vi "UI.vi"(0 "reference in":refnum<class "GUI PumpMotor.lvclass">, 5 "error in (no error)":errorcluster) -> (14 "reference out":refnum<class "GUI PumpMotor.lvclass">, 19 "error out":errorcluster)   [LabVIEW 2019, in "GUI PumpMotor.lvclass"]
uses:
  GUI PumpMotor.lvclass
  D:/GIT H4000/H4000/src/GUI_class/GUI.lvclass
  modbus engine custom/MB_ENGINE_class/Engine Alarms.ctl
  modbus engine custom/MB_ENGINE_class/Settings.ctl
  modbus engine custom/MB_ENGINE_class/cmd enum.ctl
  modbus engine custom/MB_ENGINE_class/Engine State.ctl
  TypeDef/Needle Valve Settings.ctl
  GUI_class/GUI.lvclass/GUI.ctl
  TypeDef/Needle Valve Data.ctl
  TypeDef/Needle Valve State.ctl
  modbus engine custom/MB_ENGINE_class/Limits Status.ctl
  SV_Wrap/SharedVariableWrapper.lvclass/SharedVariableWrapper.ctl
  MessageAMC_class/MessageAMC.lvclass
  D:/GIT H4000/H4000/src/MessageInterface_class/MessageInterface.lvclass
  0872259c-c1b7-4622-8eff-96544e628326.vi
  1b4fed76-272f-4eb9-b435-1b7916789d73.vi
  d0ca9bf2-7cd9-4c29-a03d-de1c10393a74.vi
  GUI_class/Set Win State.vi
  GUI_class/protected/GetSheredData.vi
  0872259c-c1b7-4622-8eff-96544e628326.vi/63923c93-3271-404a-8daf-727763f159bc.vi
  SV_Wrap/Write Var Info.vi
  SV_Wrap/Read Var Info.vi
  1b4fed76-272f-4eb9-b435-1b7916789d73.vi/fad6aa2d-1fd6-40e9-9208-cebdd25b163b.vi
  d0ca9bf2-7cd9-4c29-a03d-de1c10393a74.vi/ea186c4c-0445-4979-bfc0-5907181f2b8f.vi
  SV_Wrap/Read connection str.vi
  <userlib>/_OpenG.lib/time/time.llb/Tick Count (ms)__ogtk.vi
  GUI_class/GUI.lvclass
  MessageInterface_class/MessageInterface.lvclass
  SV_Wrap/SharedVariableWrapper.lvclass
  modbus engine custom/MB_ENGINE_class/MB_ENGINE.lvclass
panel:
  in  "Needle Valve Settings":T1={"average size"=0, "open force"=12, "close force"=12, "open settings"={"ACC Steps Per Sec^2"=0, "DEC Steps Per Sec^2"=0, "Min Velosity Step Per Sec"=0, "Max Velosity Step Per Sec"=0, "MicroStep"=0}, "close settings"={"ACC Steps Per Sec^2"=0, "DEC Steps Per Sec^2"=0, "Min Velosity Step Per Sec"=0, "Max Velosity Step Per Sec"=0, "MicroStep"=0}} caption="Settings"
  in  "Engine State":T3 items=["ACCELERATING", "DECELERATINGTOSTOP", "DECELERATING", "STEADY", "INDEX_ACCEL", "NDEX_RUN", "INDEX_DECEL", "INDEX_DWELL", "INACTIVE", "STANDBY", "STANDBYTOINACTIVE"]
  out "String 2":string
  out "String":string
  in  "clear fault":bool
  in  "stop":bool
  in  "close":bool
  in  "open":bool
  in  "Set_cmd":bool
  in  "cmd to write":T4 items=["0 Idle"=0, "1 GoTo Absolute Position"=1, "2 GoTo Relative"=2, "10 GoTo Home Position"=10, "11 Set Home Position"=11, "12 Set FindHome Mode"=12, "13 Reset FindHome Mode"=13, "14 Get FindHome State"=14, "20 Hard Stop"=20, "21 HiZ Stop"=21, "22 Soft Stop"=22, "30 Clear Fault"=30, "40 Encoder Set Home"=40, "70 Driver Init"=70]
  in  "set":bool
  out "Kinematic":T2
  out "Waveform Chart - Dark 3":dbl(graph) caption="Угол"
  out "encoder":i32(graph) caption="Энкодер"
  out "step":i32(graph) caption="ШАГ"
  out "Alarms":T5
  out "DO 19":bool
  out "Connect":bool
  in  "stop":bool
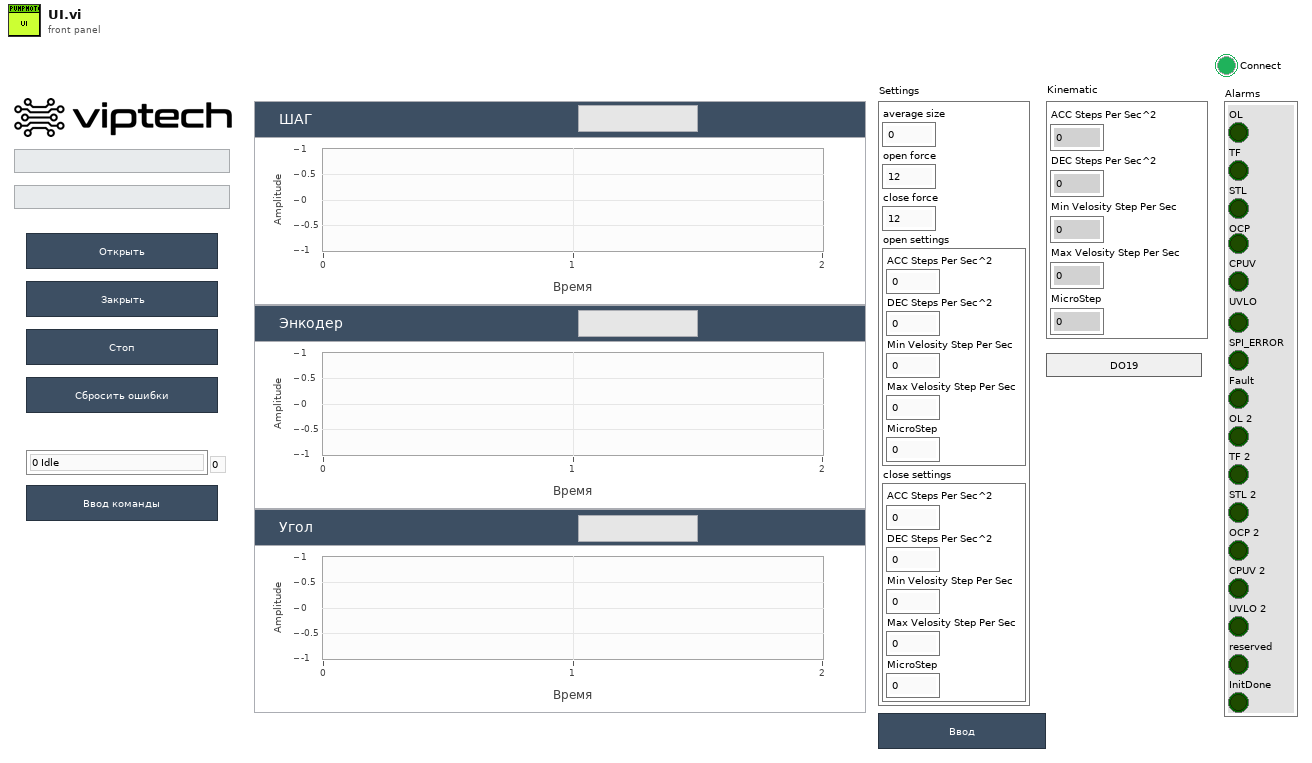
[diagram p1: front panel]
types:
  T1 = typedef "Needle Valve Settings.ctl" = cluster{"average size":i32, "open force":u16, "close force":u16, "open settings":T2, "close settings":T2}
  T2 = typedef "MB_ENGINE.lvclass/Settings.ctl" = cluster{"ACC Steps Per Sec^2":u16, "DEC Steps Per Sec^2":u16, "Min Velosity Step Per Sec":u16, "Max Velosity Step Per Sec":u16, "MicroStep":u16}
  T3 = typedef "MB_ENGINE.lvclass/Engine State.ctl" = u16
  T4 = typedef "MB_ENGINE.lvclass/cmd enum.ctl" = u16
  T5 = typedef "MB_ENGINE.lvclass/Engine Alarms.ctl" = cluster{"OL":bool, "TF":bool, "STL":bool, "OCP":bool, "CPUV":bool, "UVLO":bool, "SPI_ERROR":bool, "Fault":bool, "OL 2":bool, "TF 2":bool, "STL 2":bool, "OCP 2":bool, "CPUV 2":bool, "UVLO 2":bool, "reserved":bool, "InitDone":bool}
  T6 = enum32{"Invalid", "Standard", "Closed", "Hidden", "Minimized", "Maximized"}
  T7 = enum32{"invalid app kind", "Development System", "Run Time System", "Student Edition", "Embedded LabVIEW", "Evaluation", "Custom"}
  T8 = typedef "SharedVariableWrapper.lvclass/Config.ctl" = cluster{"connection str":string, "timeout":dbl, "ip":string}
  T9 = cluster{"Core":cluster{"Current VI Reference":refnum<vi>, "Close Panel on Exit?":bool}, "amc":refnum<class "MessageAMC.lvclass">, "satting name":string, "Needle Valve Settings":T1}
  T10 = cluster{"Current VI Reference":refnum<vi>, "Close Panel on Exit?":bool}
  T11 = typedef "Needle Valve Data.ctl" = cluster{"Engine State":T3, "StateValveModbus":T12, "Alarms":T5, "RAW Possition":i32, "Angele":dbl, "Step":i32, "Encoder":i32, "Kinematic":T2, "Limits":T13}
  T12 = typedef "Needle Valve State.ctl" = enum16{"IDLE", "OPENING", "CLOSING", "STOP"}
  T13 = typedef "MB_ENGINE.lvclass/Limits Status.ctl" = cluster{"Fault 2 Switch":bool, "Fault 1 Switch":bool, "Center(Home)":bool, "Lower Limit":bool, "Upper Limit":bool}
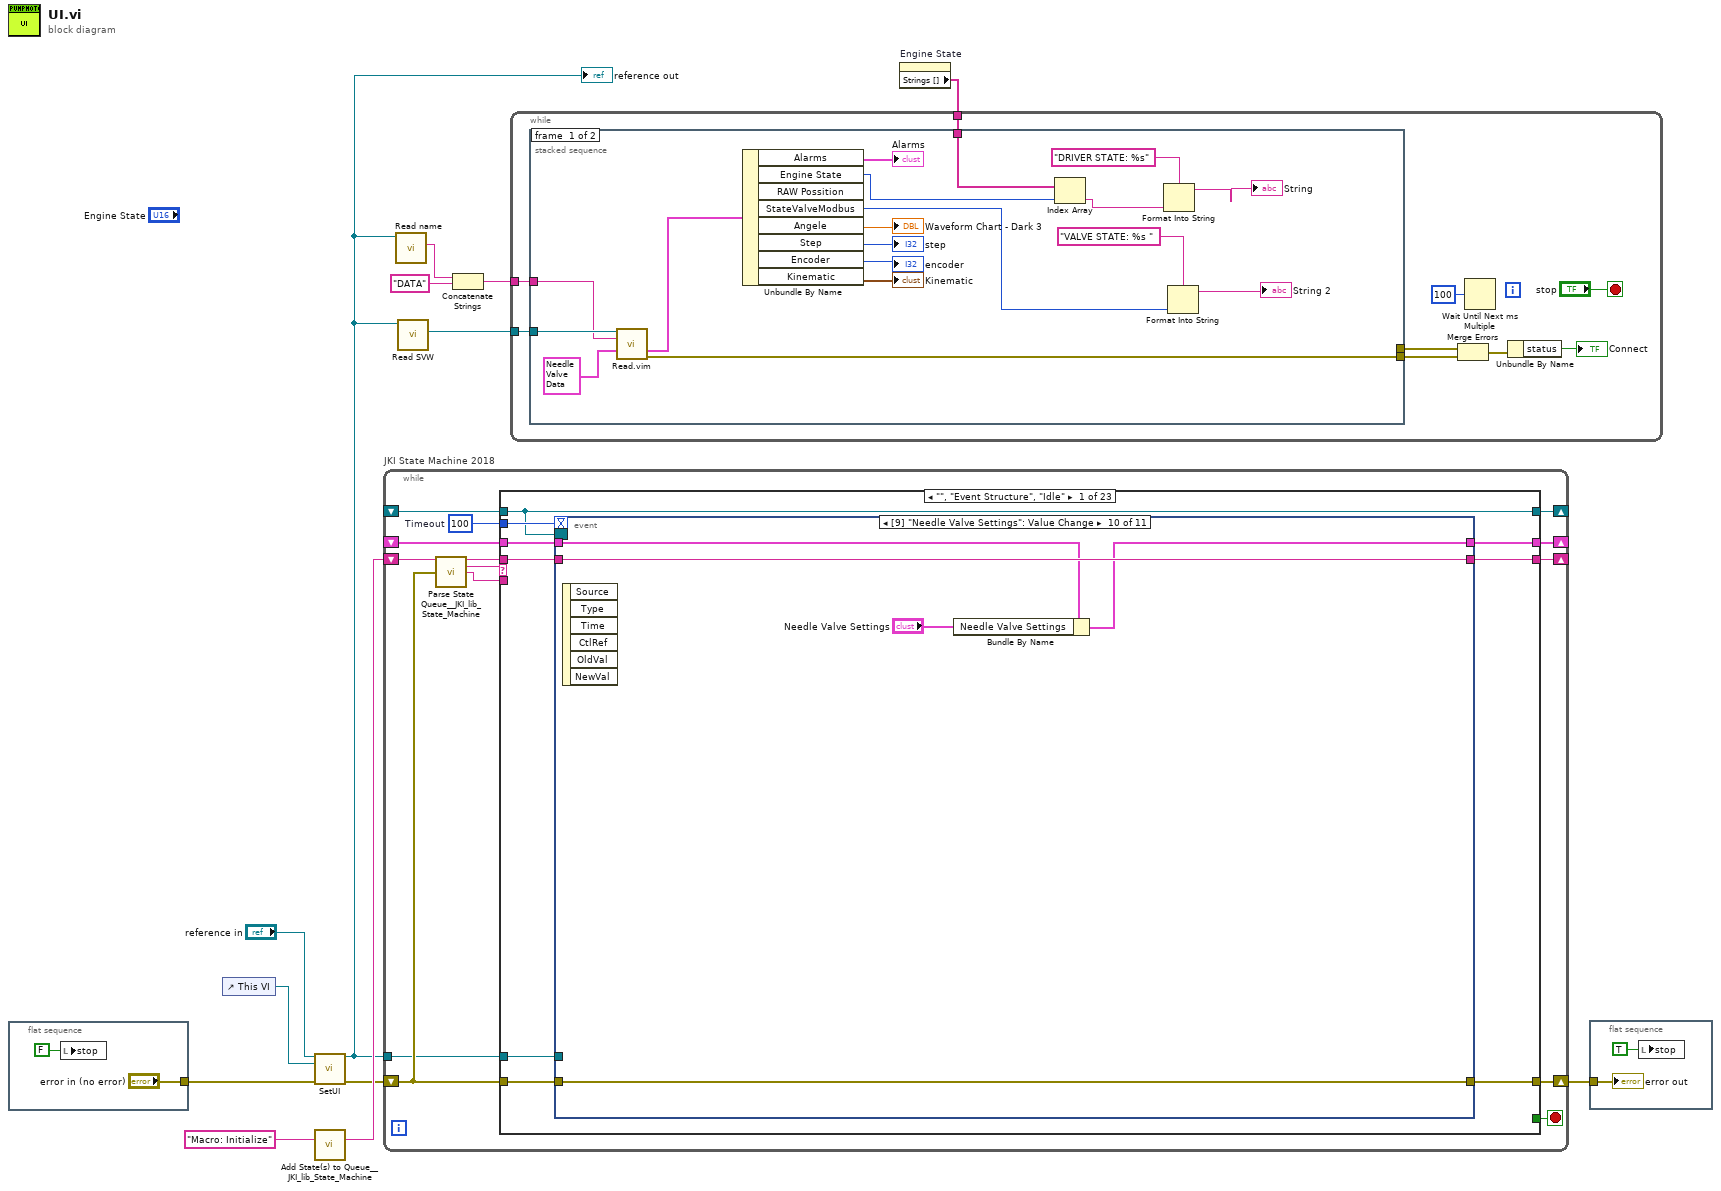
[diagram p0: block diagram]
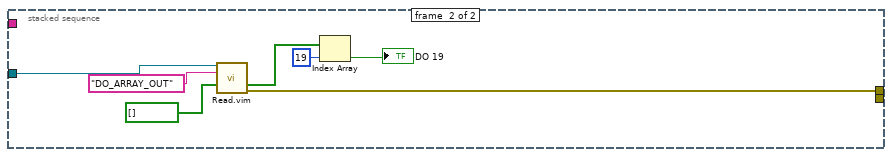
[diagram p2: hidden frame]
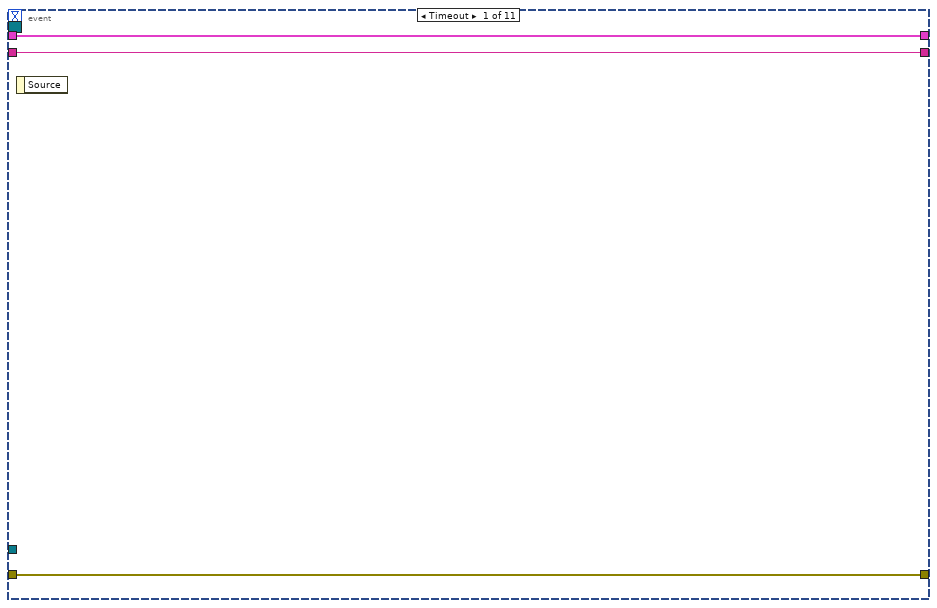
[diagram p3: hidden frame]
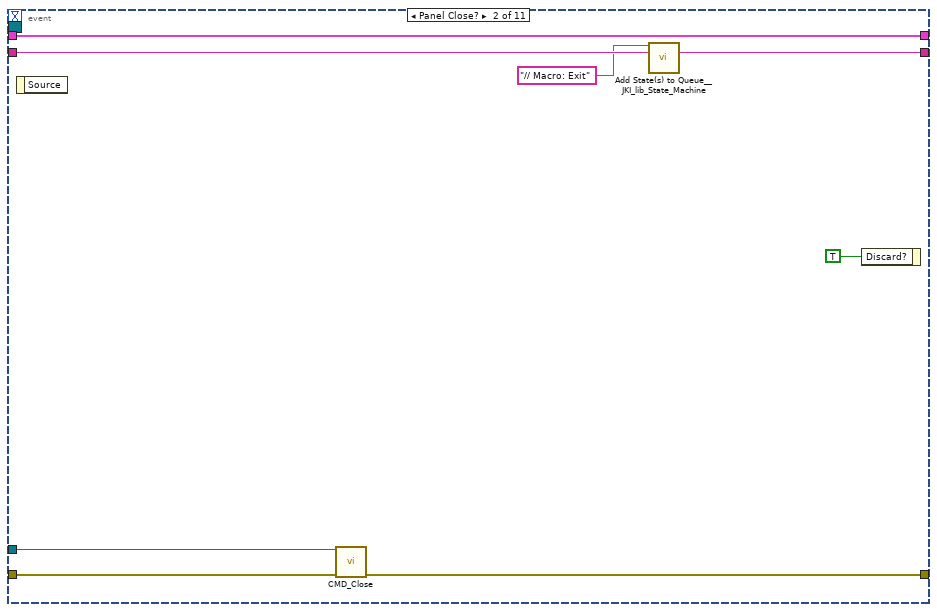
[diagram p4: hidden frame]
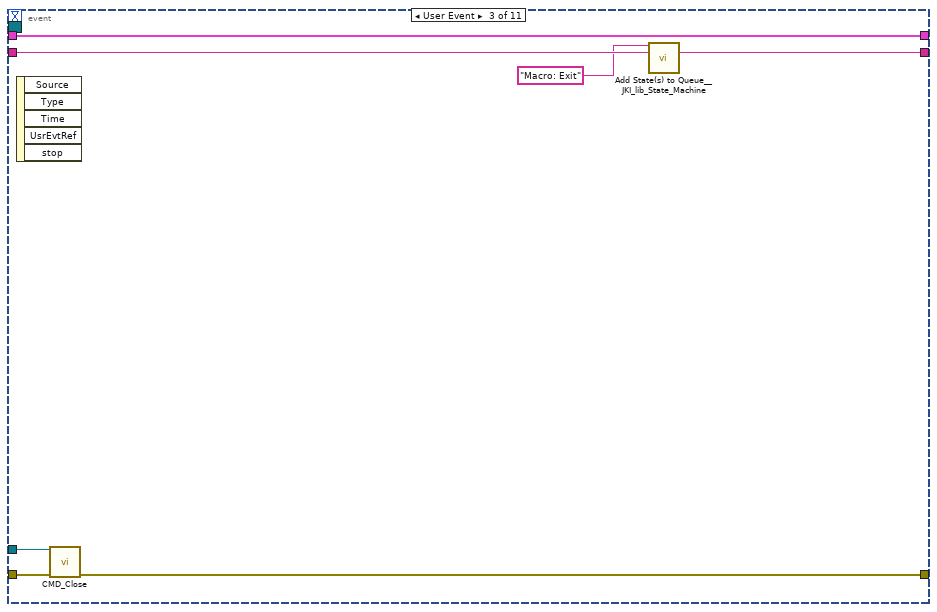
[diagram p5: hidden frame]
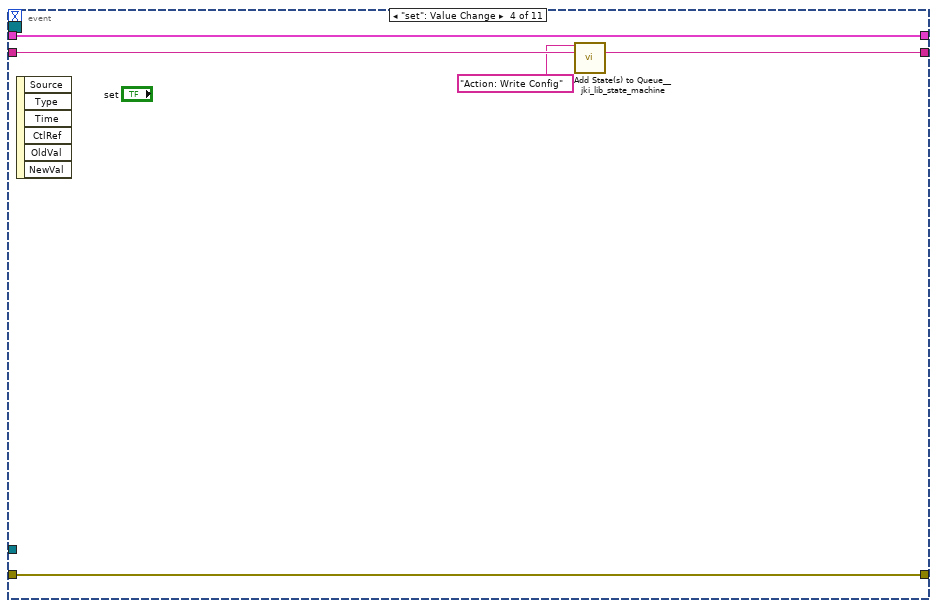
[diagram p6: hidden frame]
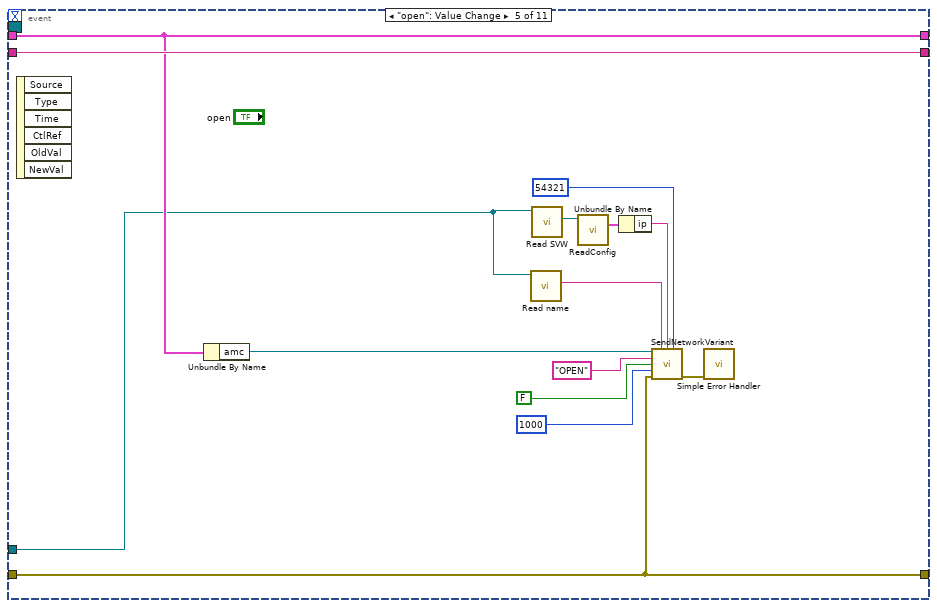
[diagram p7: hidden frame]
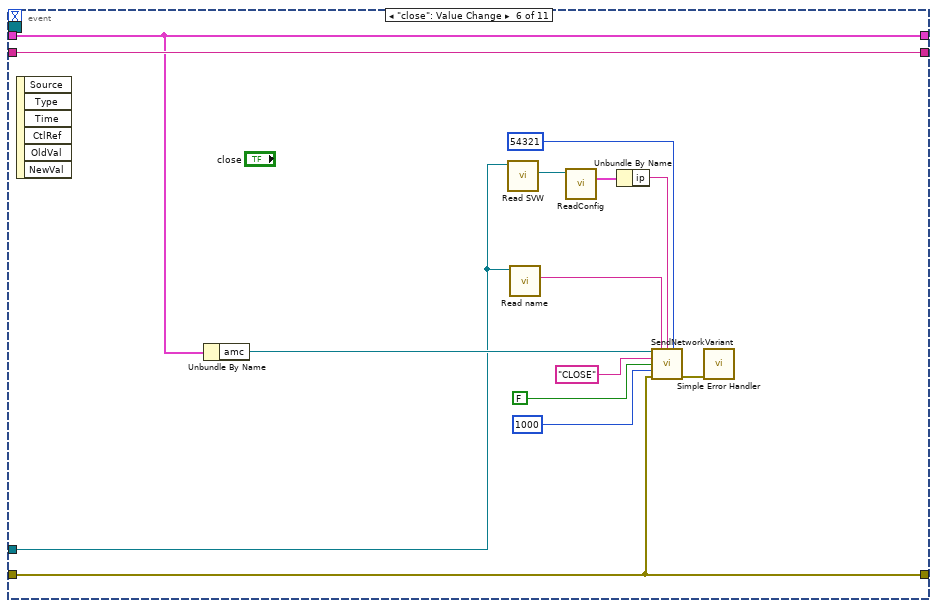
[diagram p8: hidden frame]
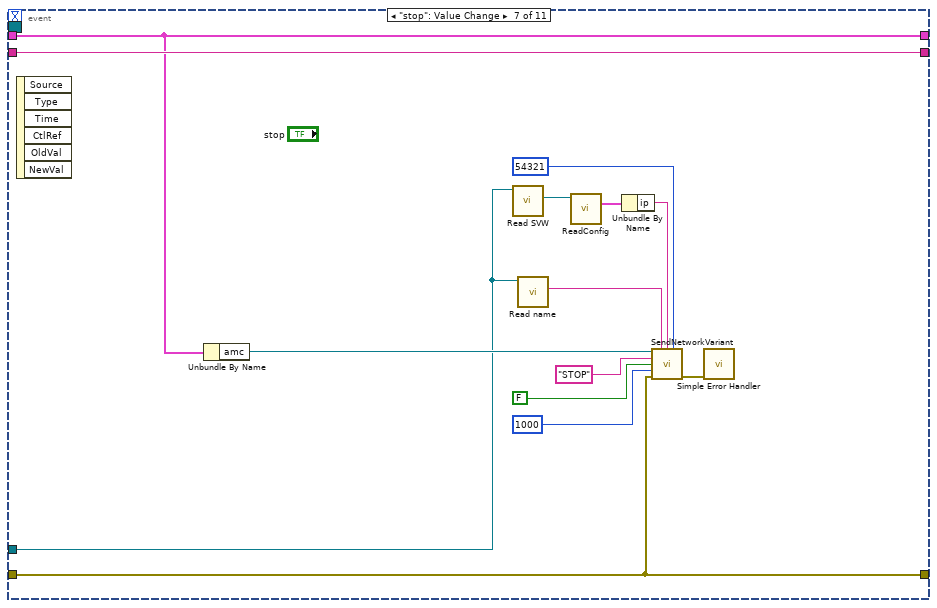
[diagram p9: hidden frame]
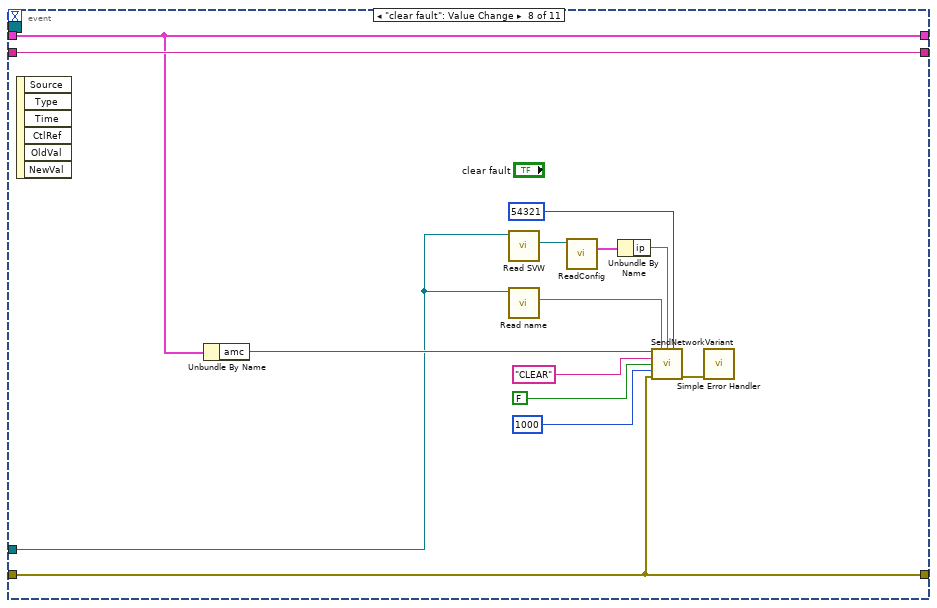
[diagram p10: hidden frame]
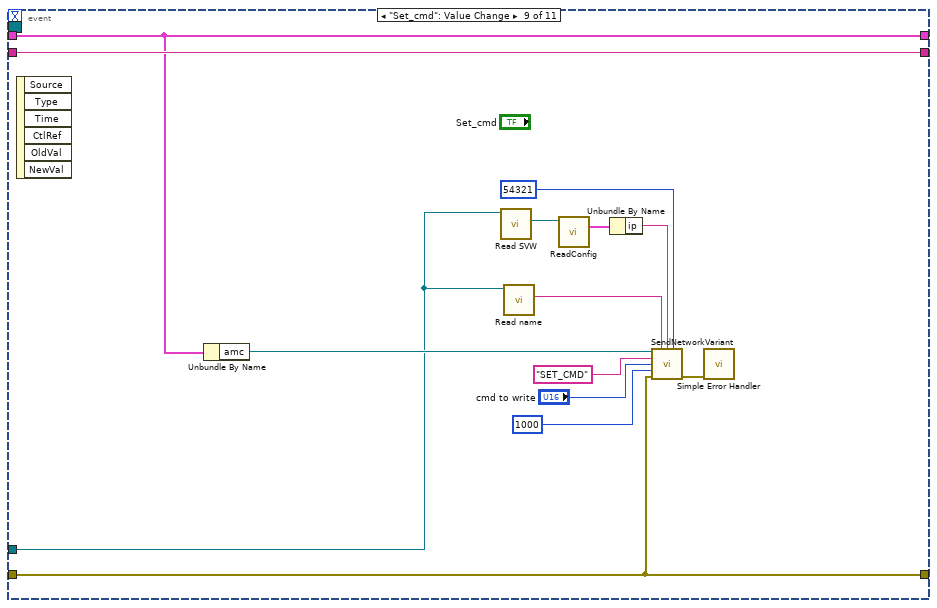
[diagram p11: hidden frame]
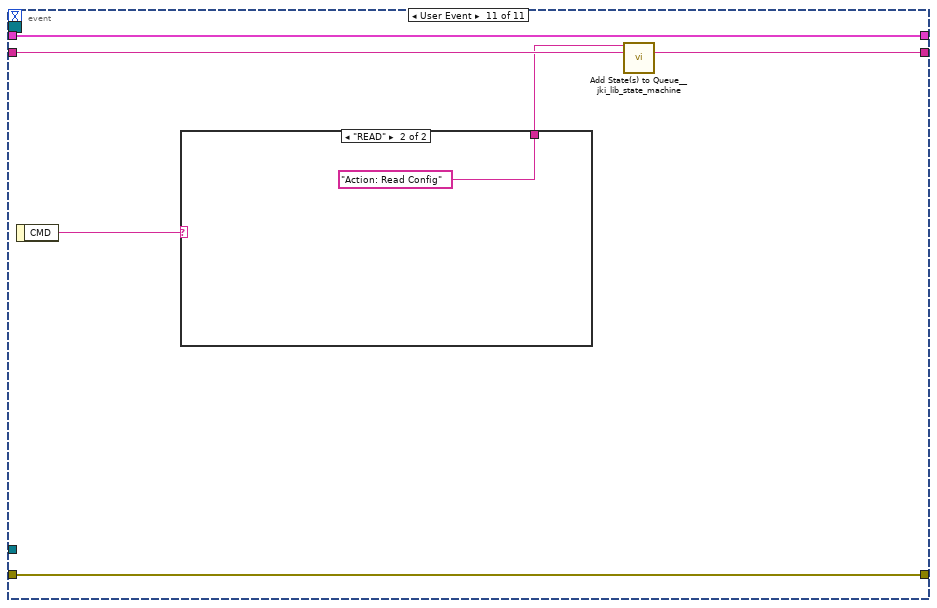
[diagram p12: hidden frame]
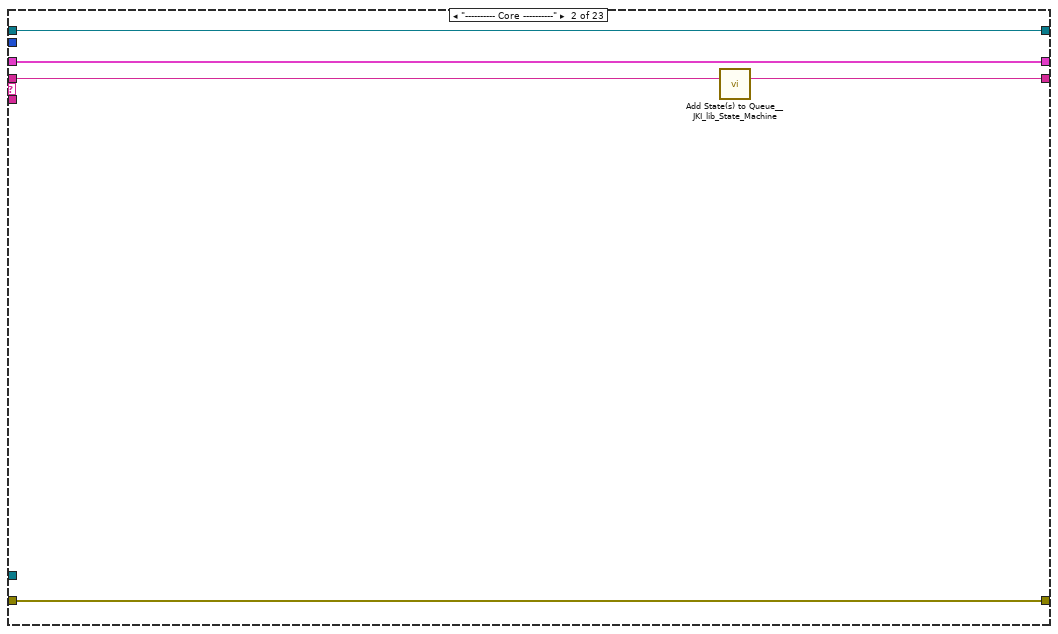
[diagram p14: hidden frame]
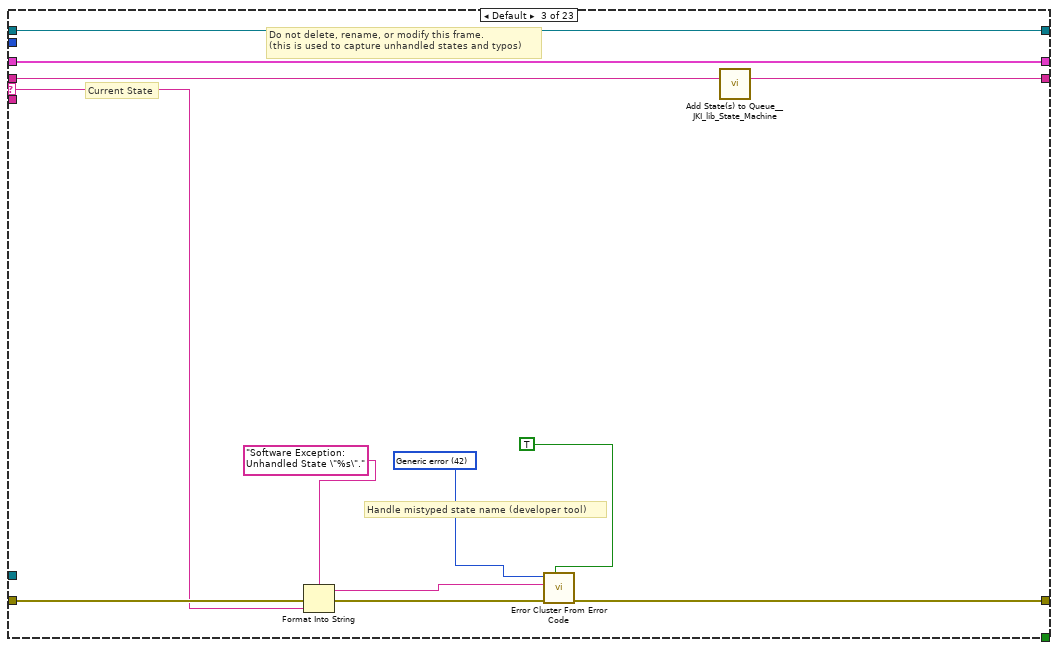
[diagram p15: hidden frame]
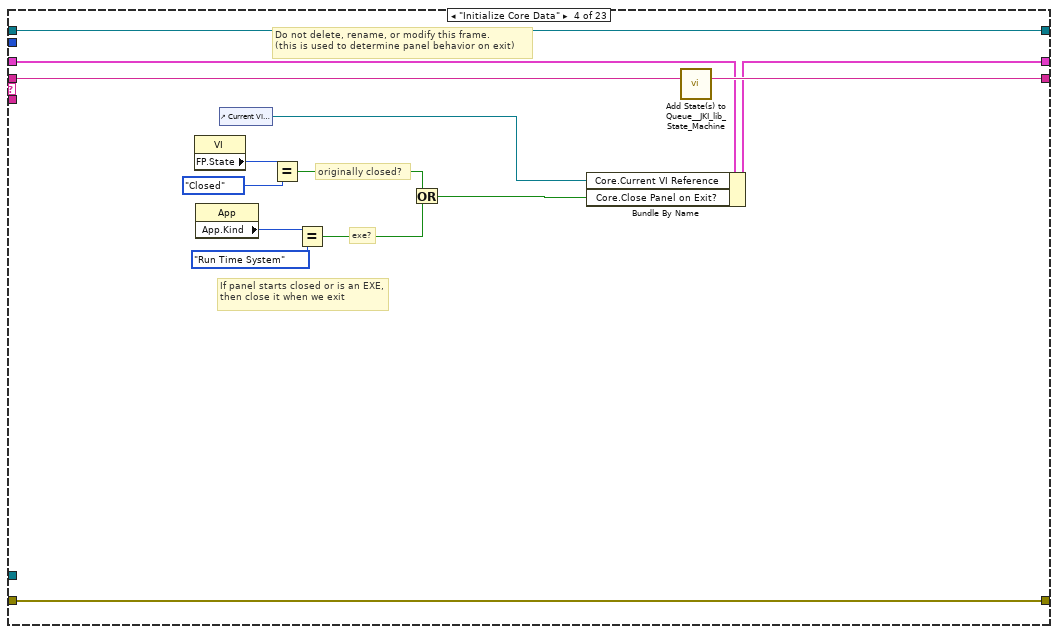
[diagram p16: hidden frame]
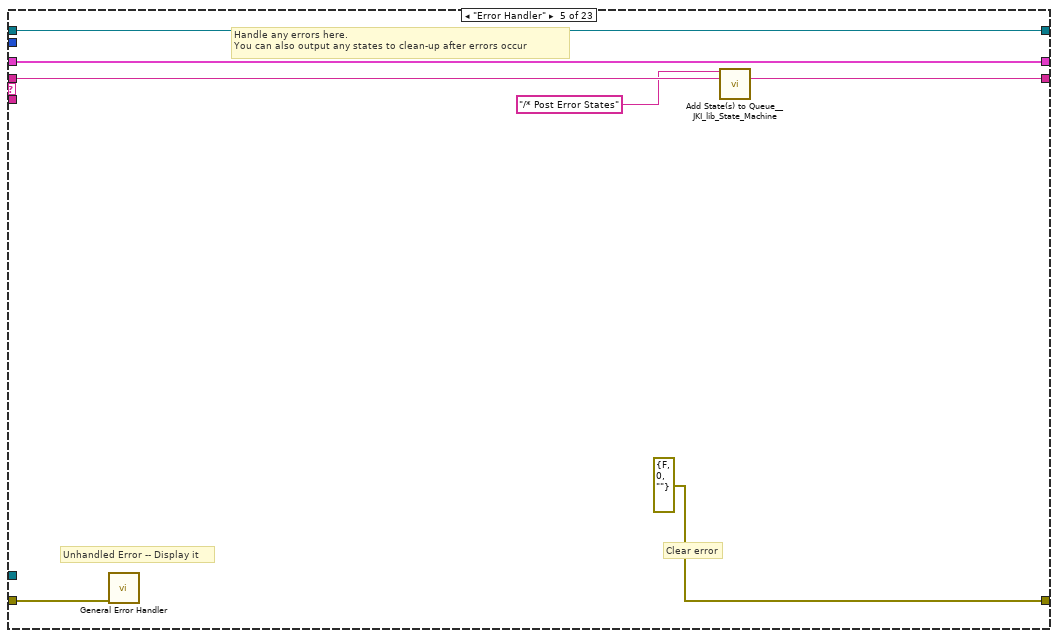
[diagram p17: hidden frame]
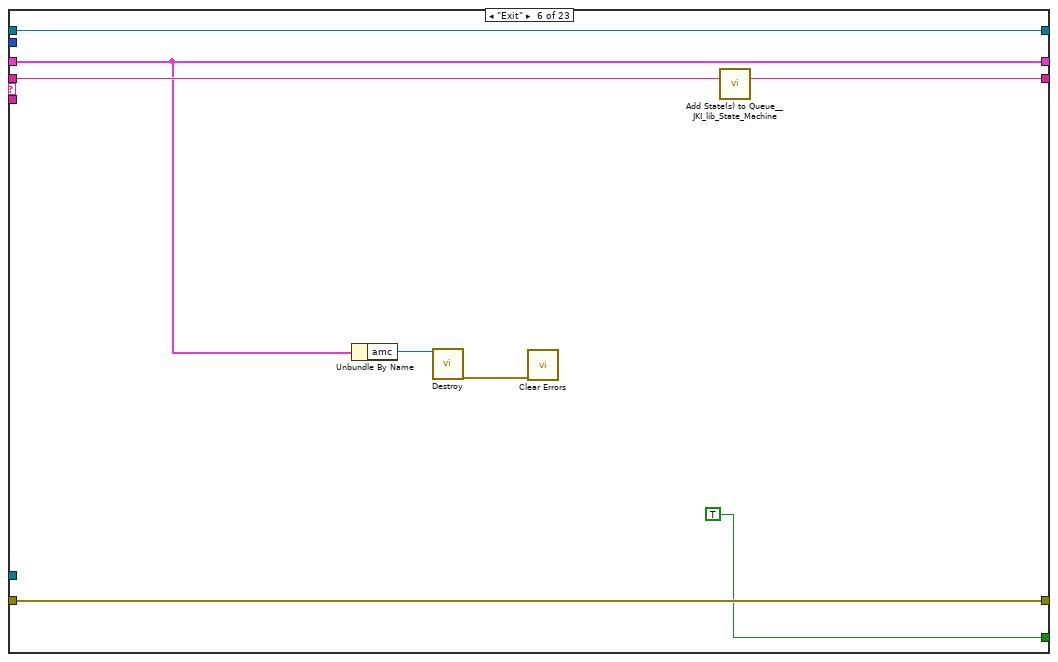
[diagram p18: hidden frame]
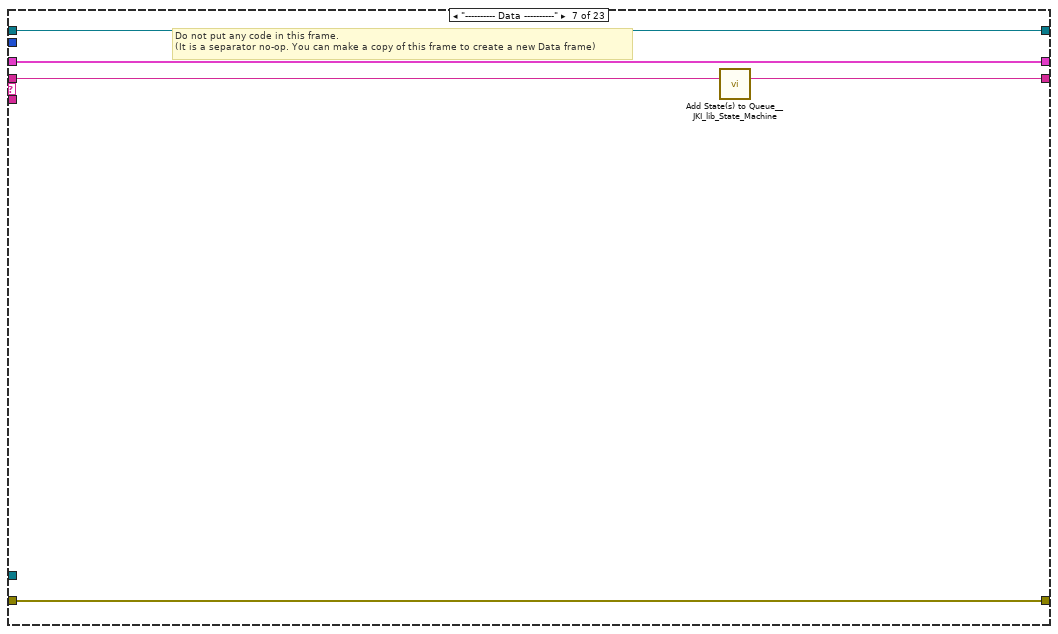
[diagram p19: hidden frame]
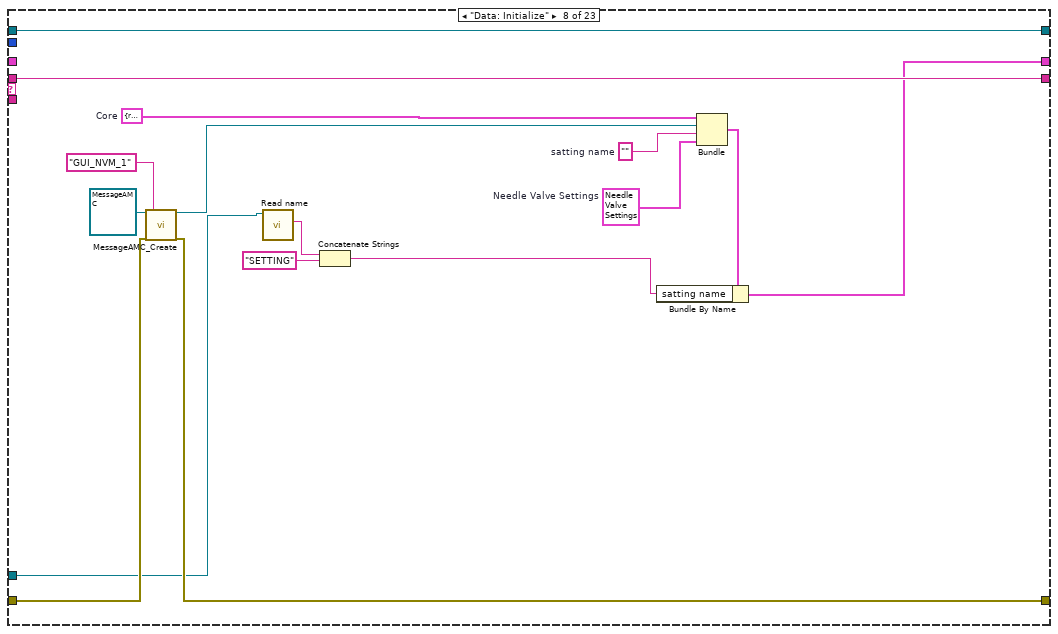
[diagram p20: hidden frame]
diagram:
  n1 = flat-sequence {
    tunnel: ["error in (no error)"] -> w10
    frame #0 {
      n2 = local write "stop"(FALSE ("stop")) -> ()
    }
  }
  n3 = control-ref of="This VI"() -> (w8:refnum<vi>)
  n4 = call "SetUI.vi"("reference in"="reference in", "UI VI"=w8, "error in (no error)"=w10) -> ("reference out"=w4:refnum<class "GUI PumpMotor.lvclass">, "error out"=w7:errorcluster)  [unwired: 11 in]
  "reference out" <- w4
  n5 = call <vilib>:"Add State(s) to Queue__JKI_lib_State_Machine.vi"("State(s) in (\"\")"="Macro: Initialize") -> ("States Out"=w13:string)  [unwired: 14 in]
  n6 = while "JKI State Machine 2018" {
    shift-right: [w22] -> _
    shift-left: _ -> [w21]
    shift-right: [w25] -> w11
    shift-left: w7 -> [w19]
    shift-right: [w24] -> _
    shift-left: w13 -> [w26]
    tunnel: w4 -> [w18]
    shift-right: [w17] -> _
    shift-left: _ -> [w16]
    stop <- w23 stop-if-true
    w20 = 100  # Timeout
    n7 = call <vilib>:"Parse State Queue__JKI_lib_State_Machine.vi"("State Queue"=w26, "Error In (no error)"=w19) -> ("Remaining States"=w28:string, "Current State"=w29:string, "Arguments"=w27:string)  [unwired: 11 in]
    n8 = case shown="\"\", \"Event Structure\", \"Idle\"" w29 {
      selector: w29 -> [_ _ w150 _ _ _ _ _ _ _ _ _ _ _ _ _ _ _ _ _ _ _ _]
      tunnel: w28 -> [w38 w148 w154 w174 w181 w189 w194 w210 w217 w222 w230 w236 w241 w245 w252 w264 w334 w340 w346 w358 w362 w365 w392]
      tunnel: w27 -> [_ _ _ _ _ _ _ _ _ _ _ _ _ _ w247 w258 _ _ _ _ _ _ _]
      tunnel: w21 -> [w36 w145 w152 w167 w178 w184 w191 _ w212 w219 w229 w234 w238 w244 w250 w260 w331 w337 w343 w355 w360 w367 w380]
      tunnel: [w35 w146 w156 w171 errorcluster {"status"=FALSE, "code"=0, "source"=""} ("error out") w187 w192 w203 w213 w220 w227 w231 w239 w243 w248 w261 w332 w338 w344 w356 w361 w368 w381] -> w25
      tunnel: w19 -> [w34 w146 w155 w171 w177 w187 w192 w204 w214 w220 w226 w232 w239 w243 w249 w262 w332 w338 w344 w356 w361 w369 w382]
      tunnel: [w37 w147 w153 w173 w180 w188 w193 w210 w216 w221 w230 w235 w240 w245 w251 w263 w333 w339 w345 w357 w362 w365 w392] -> w24
      tunnel: [_ _ _ _ _ TRUE _ _ _ _ _ _ _ _ _ _ _ _ _ _ _ _ _] -> w23
      tunnel: [w33 w145 w152 w172 w178 w184 w191 w196 w212 w219 w229 w234 w238 w244 w250 w260 w331 w337 w343 w355 w360 w366 w380] -> w22
      tunnel: w20 -> [w32 _ _ _ _ _ _ _ _ _ _ _ _ _ _ _ _ _ _ _ _ _ _]
      tunnel: w18 -> [w31 _ _ _ _ _ _ w199 _ _ w225 _ _ _ _ _ _ _ _ _ _ w364 w377]
      tunnel: [w30 w144 w149 w161 w175 w185 w190 w207 w211 w218 w228 w233 w237 w242 w246 w257 w330 w335 w341 w348 w359 w370 w391] -> w17
      tunnel: w16 -> [w30 w144 w149 w161 w175 w185 w190 w207 w211 w218 _ w233 w237 w242 w246 w257 w330 w335 w341 w348 w359 w370 w391]
      frame "", "Event Structure", "Idle" {
        n9 = event shown="[9] \"Needle Valve Settings\": Value Change" {
          selector: w30 -> [_ _ _ _ _ _ _ _ _ _ _]
          dyn-events: _ -> [_ _ _ _ _ _ _ _ _ _ _]
          timeout: w32 -> [_ _ _ _ _ _ _ _ _ _ _]
          tunnel: w38 -> [w41 w49 w56 w58 w75 w89 w103 w117 w131 w136 w139]
          tunnel: [w41 w48 w55 w59 w75 w89 w103 w117 w131 w136 w140] -> w37
          tunnel: w36 -> [w39 w47 w54 w60 w69 w83 w97 w111 w125 w134 w141]
          tunnel: [w40 w42 w50 w61 w64 w78 w92 w106 w121 w135 w142] -> w35
          tunnel: w34 -> [w40 w43 w51 w61 w64 w78 w92 w106 w121 w135 w142]
          tunnel: [w39 w47 w54 w60 w69 w83 w97 w111 w125 w133 w141] -> w33
          tunnel: w31 -> [_ w44 w52 _ w62 w77 w91 w105 w119 _ _]
          event Timeout {
            n10 = event-data() -> ()  [unwired: 1 in, 1 out]
          }
          event Panel Close? {
            n11 = event-data() -> ()  [unwired: 1 in, 1 out]
            n12 = call "CMD_Close.vi"("reference in"=w44, "error in (no error)"=w43) -> ("error out"=w42:errorcluster)  [unwired: 12 in, 1 out]
            n13 = call <vilib>:"Add State(s) to Queue__JKI_lib_State_Machine.vi"("State(s) in Front (\"\")"="// Macro: Exit", "State(s) in (\"\")"=w49) -> ("States Out"=w48:string)  [unwired: 13 in]
            n14 = event-data("Discard?"=TRUE) -> ()  [unwired: 1 in, 1 out]
          }
          event User Event {
            n15 = event-data() -> ()  [unwired: 1 in, 5 out]
            n16 = call "CMD_Close.vi"("reference in"=w52, "error in (no error)"=w51) -> ("error out"=w50:errorcluster)  [unwired: 12 in, 1 out]
            n17 = call <vilib>:"Add State(s) to Queue__JKI_lib_State_Machine.vi"("State(s) in Front (\"\")"="Macro: Exit", "State(s) in (\"\")"=w56) -> ("States Out"=w55:string)  [unwired: 13 in]
          }
          event "set": Value Change {
            n18 = event-data() -> ()  [unwired: 1 in, 6 out]
            n19 = call <vilib>:"Add State(s) to Queue__jki_lib_state_machine.vi"("State(s) in Front (\"\")"="Action: Write Config" ("State(s) in Front (\"\")"), "State(s) in (\"\")"=w58) -> ("States Out"=w59:string)  [unwired: 13 in]
          }
          event "open": Value Change {
            n20 = event-data() -> ()  [unwired: 1 in, 6 out]
            n21 = Unbundle By Name(w69) -> ("amc"=w68:refnum<class "MessageAMC.lvclass">)
            n22 = call "Read name.vi"("GUI in"=w62) -> ("name"=w63:string)  [unwired: 9 in, 1 out]
            n23 = call "Read SVW.vi"("GUI in"=w62) -> ("SharedVariableWrapper.lvclass"=w71:refnum<class "SharedVariableWrapper.lvclass">)  [unwired: 10 in]
            n24 = call "ReadConfig.vi"("SharedVariableWrapper in"=w71) -> ("config"=w70:T8)  [unwired: 12 in, 2 out]
            n25 = Unbundle By Name(w70) -> ("ip"=w67:string)
            n26 = call "SendNetworkVariant.vi"("reference in"=w68, "receiver process"=w63, "receiver host"=w67, "receiver port (0)"=u16 54321, "name"="OPEN", "data"=FALSE, "timeout (25000 ms)"=1000, "error in (no error)"=w64) -> ("error out"=w65:errorcluster)  [unwired: 5 in, 2 out]
            n27 = call <vilib>:"Simple Error Handler.vi"("error in (no error)"=w65) -> ()  [unwired: 4 in, 5 out]
          }
          event "close": Value Change {
            n28 = event-data() -> ()  [unwired: 1 in, 6 out]
            n29 = Unbundle By Name(w83) -> ("amc"=w82:refnum<class "MessageAMC.lvclass">)
            n30 = call "Read SVW.vi"("GUI in"=w77) -> ("SharedVariableWrapper.lvclass"=w85:refnum<class "SharedVariableWrapper.lvclass">)  [unwired: 10 in]
            n31 = call "Read name.vi"("GUI in"=w77) -> ("name"=w76:string)  [unwired: 9 in, 1 out]
            n32 = call "ReadConfig.vi"("SharedVariableWrapper in"=w85) -> ("config"=w84:T8)  [unwired: 12 in, 2 out]
            n33 = Unbundle By Name(w84) -> ("ip"=w81:string)
            n34 = call "SendNetworkVariant.vi"("reference in"=w82, "receiver process"=w76, "receiver host"=w81, "receiver port (0)"=u16 54321, "name"="CLOSE", "data"=FALSE, "timeout (25000 ms)"=1000, "error in (no error)"=w78) -> ("error out"=w79:errorcluster)  [unwired: 5 in, 2 out]
            n35 = call <vilib>:"Simple Error Handler.vi"("error in (no error)"=w79) -> ()  [unwired: 4 in, 5 out]
          }
          event "stop": Value Change {
            n36 = event-data() -> ()  [unwired: 1 in, 6 out]
            n37 = Unbundle By Name(w97) -> ("amc"=w96:refnum<class "MessageAMC.lvclass">)
            n38 = call "Read SVW.vi"("GUI in"=w91) -> ("SharedVariableWrapper.lvclass"=w99:refnum<class "SharedVariableWrapper.lvclass">)  [unwired: 10 in]
            n39 = call "Read name.vi"("GUI in"=w91) -> ("name"=w90:string)  [unwired: 9 in, 1 out]
            n40 = call "ReadConfig.vi"("SharedVariableWrapper in"=w99) -> ("config"=w98:T8)  [unwired: 12 in, 2 out]
            n41 = Unbundle By Name(w98) -> ("ip"=w95:string)
            n42 = call "SendNetworkVariant.vi"("reference in"=w96, "receiver process"=w90, "receiver host"=w95, "receiver port (0)"=u16 54321, "name"="STOP", "data"=FALSE, "timeout (25000 ms)"=1000, "error in (no error)"=w92) -> ("error out"=w93:errorcluster)  [unwired: 5 in, 2 out]
            n43 = call <vilib>:"Simple Error Handler.vi"("error in (no error)"=w93) -> ()  [unwired: 4 in, 5 out]
          }
          event "clear fault": Value Change {
            n44 = event-data() -> ()  [unwired: 1 in, 6 out]
            n45 = Unbundle By Name(w111) -> ("amc"=w110:refnum<class "MessageAMC.lvclass">)
            n46 = call "Read SVW.vi"("GUI in"=w105) -> ("SharedVariableWrapper.lvclass"=w113:refnum<class "SharedVariableWrapper.lvclass">)  [unwired: 10 in]
            n47 = call "Read name.vi"("GUI in"=w105) -> ("name"=w104:string)  [unwired: 9 in, 1 out]
            n48 = call "ReadConfig.vi"("SharedVariableWrapper in"=w113) -> ("config"=w112:T8)  [unwired: 12 in, 2 out]
            n49 = Unbundle By Name(w112) -> ("ip"=w109:string)
            n50 = call "SendNetworkVariant.vi"("reference in"=w110, "receiver process"=w104, "receiver host"=w109, "receiver port (0)"=u16 54321, "name"="CLEAR", "data"=FALSE, "timeout (25000 ms)"=1000, "error in (no error)"=w106) -> ("error out"=w107:errorcluster)  [unwired: 5 in, 2 out]
            n51 = call <vilib>:"Simple Error Handler.vi"("error in (no error)"=w107) -> ()  [unwired: 4 in, 5 out]
          }
          event "Set_cmd": Value Change {
            n52 = event-data() -> ()  [unwired: 1 in, 6 out]
            n53 = Unbundle By Name(w125) -> ("amc"=w124:refnum<class "MessageAMC.lvclass">)
            n54 = call "Read SVW.vi"("GUI in"=w119) -> ("SharedVariableWrapper.lvclass"=w127:refnum<class "SharedVariableWrapper.lvclass">)  [unwired: 10 in]
            n55 = call "Read name.vi"("GUI in"=w119) -> ("name"=w118:string)  [unwired: 9 in, 1 out]
            n56 = call "ReadConfig.vi"("SharedVariableWrapper in"=w127) -> ("config"=w126:T8)  [unwired: 12 in, 2 out]
            n57 = Unbundle By Name(w126) -> ("ip"=w123:string)
            n58 = call "SendNetworkVariant.vi"("reference in"=w124, "receiver process"=w118, "receiver host"=w123, "receiver port (0)"=u16 54321, "name"="SET_CMD", "data"="cmd to write", "timeout (25000 ms)"=1000, "error in (no error)"=w121) -> ("error out"=w122:errorcluster)  [unwired: 5 in, 2 out]
            n59 = call <vilib>:"Simple Error Handler.vi"("error in (no error)"=w122) -> ()  [unwired: 4 in, 5 out]
          }
          event Value Change {
            n60 = event-data() -> ()  [unwired: 1 in, 6 out]
            n61 = Bundle By Name(cluster=w134, "Needle Valve Settings"="Needle Valve Settings") -> (w133:T9)
          }
          event User Event {
            n62 = event-data() -> ("CMD"=w138:string)  [unwired: 1 in]
            n63 = case shown="\"READ\"" w138 {
              tunnel: [_ "Action: Read Config" ("State(s) in Front (\"\")")] -> w137
              frame "False", Default {
              }
              frame "READ" {
              }
            }
            n64 = call <vilib>:"Add State(s) to Queue__jki_lib_state_machine.vi"("State(s) in Front (\"\")"=w137, "State(s) in (\"\")"=w139) -> ("States Out"=w140:string)  [unwired: 13 in]
          }
        }
      }
      frame "---------- Core ----------" {
        n65 = call <vilib>:"Add State(s) to Queue__JKI_lib_State_Machine.vi"("State(s) in (\"\")"=w148) -> ("States Out"=w147:string)  [unwired: 14 in]
      }
      frame Default {
        w159 = 42 items=["No error", "Argument error", "Memory is full", "Out of zone", "End of file", "File already open", "Generic file I/O error", "File not found", "File permission error", "Disk is full", "Duplicate path", "Too many files open", "System feature not enabled", "Resource file not found", "Cannot add resource", "Resource not found", "Image not found", "Image memory error", "Pen does not exist", "Config type invalid", "Config token not found", "Config parse error", "Config memory error", "Bad external code format", "Bad external code offset", "External code not present", "Null window", "Destroy window error", "Null menu", "Print aborted", "Bad print record", "Print driver error", "Windows error during printing", "Memory error during printing", "Print dialog error", "Generic print error", "Invalid device refnum", "Device not found", "Device parameter error", "Device unit error", "Cannot open device", "Device call aborted", "Generic error", "Cancelled by user", "Object ID too low", "Object ID too high", "Object not in heap", "Unknown heap", "Unknown object (invalid DefProc)", "Unknown object (DefProc not in table)", "Message out of range", "Invalid (null) method", "Unknown message", "Manager call not supported", "Bad address", "Network operation in progress", "Network operation timed out", "Connection is busy", "Network attribute not supported", "Network error", "Address in use", "System out of memory", "Connection aborted", "Connection refused", "Not connected", "Already connected", "Connection closed", "Initialization error (interapplication manager)", "Bad occurrence", "Wait on unbound occurrence handler", "Occurrence queue overflow", "Datalog type conflict", "Unused", "Unrecognized type (interapplication manager)", "Memory corrupt", "Failed to make temporary DLL", "Old CIN version", "Drag socket not found", "Failed to load drop-object", "Failed to register OLE object", "Failed to release OLE object", "Format specifier type mismatch", "Unknown format specifier", "Too few format specifiers", "Too many format specifiers", "Scan failed", "Newer CIN version", "Error converting to variant", "Runtime menu error", "Password tampered", "Variant attribute not found", "Incompatible variant data type", "Event data is not available", "Event Store is not present", "Occurrence is not found", "Event Queue is not created", "Event info is not available", "Refnum passed is NULL", "Error retrieving Class GUID", "Error retrieving CoClass GUID", "Error retrieving TypeLib GUID.", "Bad built application magic bytes.", "Specific driver is different from the specific driver associated with the Logical Name.", "There is no session opened to the class driver.", "Max Error", "MAX - Error with config objects", "MAX - Error loading configuration", "MAX - Group not supported"]
        # "Current State"
        # "Do not delete, rename, or modify this frame.\n(this is used to capture unhandled states and typos)"
        # "Handle mistyped state name (developer tool)"
        n66 = Format Into String(format string="Software Exception: Unhandled State \"%s\"." ("message"), error in=w155, w150) -> (resulting string=w158:string, error out=w157:errorcluster)  [unwired: 1 in]
        n67 = call <vilib>:"Error Cluster From Error Code.vi"("show call chain? (False)"=TRUE, "error in (no error)"=w157, "error message (\"\")"=w158, "error code (0)"=w159) -> ("error out"=w156:errorcluster)  [unwired: 5 in]
        n68 = call <vilib>:"Add State(s) to Queue__JKI_lib_State_Machine.vi"("State(s) in (\"\")"=w154) -> ("States Out"=w153:string)  [unwired: 14 in]
      }
      frame "Initialize Core Data" {
        # "Do not delete, rename, or modify this frame.\n(this is used to determine panel behavior on exit)"
        # "originally closed?"
        # "exe?"
        # "If panel starts closed or is an EXE, then close it when we exit"
        n69 = property class="VI"() -> ("FP.State"=w164:T6)  [unwired: 2 in, 2 out]
        n70 = property class="App"() -> ("App.Kind"=w170:T7)  [unwired: 2 in, 2 out]
        n71 = control-ref of="Current VI Reference"() -> (w165:refnum<vi>)
        n72 = Equal?(x=w164, y=T6."Closed" ("Front Panel Window:State")) -> (x = y?=w162:bool)
        n73 = Equal?(x=w170, y=T7."Run Time System" ("Application:Kind")) -> (x = y?=w168:bool)
        n74 = Or(x=w162, y=w168) -> (x .or. y?=w166:bool)
        n75 = Bundle By Name(cluster=w167, "Core.Current VI Reference"=w165, "Core.Close Panel on Exit?"=w166) -> (w172:T9)
        n76 = call <vilib>:"Add State(s) to Queue__JKI_lib_State_Machine.vi"("State(s) in (\"\")"=w174) -> ("States Out"=w173:string)  [unwired: 14 in]
      }
      frame "Error Handler" {
        # "Unhandled Error -- Display it"
        # "Handle any errors here.\nYou can also output any states to clean-up after errors occur"
        # "Clear error"
        n77 = call <vilib>:"General Error Handler.vi"("error in (no error)"=w177) -> ()  [unwired: 10 in, 5 out]
        n78 = call <vilib>:"Add State(s) to Queue__JKI_lib_State_Machine.vi"("State(s) in Front (\"\")"="/* Post Error States", "State(s) in (\"\")"=w181) -> ("States Out"=w180:string)  [unwired: 13 in]
      }
      frame "Exit" {
        n79 = Unbundle By Name(w184) -> ("amc"=w183:refnum<class "MessageAMC.lvclass">)
        n80 = call-dynamic "Destroy.vi"("reference in"=w183) -> ("error out"=w182:errorcluster)  [unwired: 17 in, 1 out]
        n81 = call <vilib>:"Clear Errors.vi"("error in (no error)"=w182) -> ()  [unwired: 5 in, 2 out]
        n82 = call <vilib>:"Add State(s) to Queue__JKI_lib_State_Machine.vi"("State(s) in (\"\")"=w189) -> ("States Out"=w188:string)  [unwired: 14 in]
      }
      frame "---------- Data ----------" {
        # "Do not put any code in this frame.\n(It is a separator no-op. You can make a copy of this frame to create a new Data frame)"
        n83 = call <vilib>:"Add State(s) to Queue__JKI_lib_State_Machine.vi"("State(s) in (\"\")"=w194) -> ("States Out"=w193:string)  [unwired: 14 in]
      }
      frame "Data: Initialize" {
        w197 = ""  # satting name
        w201 = T1 {"average size"=0, "open force"=12, "close force"=12, "open settings"={"ACC Steps Per Sec^2"=0, "DEC Steps Per Sec^2"=0, "Min Velosity Step Per Sec"=0, "Max Velosity Step Per Sec"=0, "MicroStep"=0}, "close settings"={"ACC Steps Per Sec^2"=0, "DEC Steps Per Sec^2"=0, "Min Velosity Step Per Sec"=0, "Max Velosity Step Per Sec"=0, "MicroStep"=0}}  # Needle Valve Settings
        w208 = T10 {"Current VI Reference"=refnum, "Close Panel on Exit?"=FALSE}  # Core
        n84 = call "MessageAMC_Create.vi"("reference in"=refnum<class "MessageAMC.lvclass"> refnum, "error in (no error)"=w204, "message queue name"="GUI_NVM_1") -> ("amc"=w205:refnum<class "MessageAMC.lvclass">, "error out"=w203:errorcluster)  [unwired: 15 in]
        n85 = call "Read name.vi"("GUI in"=w199) -> ("name"=w200:string)  [unwired: 9 in, 1 out]
        n86 = Concatenate Strings(w200, "SETTING" ("name")) -> (w195:string)
        n87 = Bundle("Core"=w208, "amc"=w205, "satting name"=w197, "Needle Valve Settings"=w201) -> (w209:T9)  [unwired: 1 in]
        n88 = Bundle By Name(cluster=w209, "satting name"=w195) -> (w196:T9)
      }
      frame "Data: Cleanup" {
        # "Cleanup any data and references, here.\n(this is called automatically, by the Macro: Exit)"
        n89 = Unbundle By Name(w212) -> ("Core.Current VI Reference"=w215:refnum<vi>)
        n90 = Close Reference(reference=w215, error in (no error)=w214) -> (error out=w213:errorcluster)
        n91 = call <vilib>:"Add State(s) to Queue__JKI_lib_State_Machine.vi"("State(s) in (\"\")"=w217) -> ("States Out"=w216:string)  [unwired: 14 in]
      }
      frame "---------- Events ----------" {
        # "Do not put any code in this frame.\n(It is a separator no-op. You can make a copy of this frame to create a new UI frame)"
        n92 = call <vilib>:"Add State(s) to Queue__JKI_lib_State_Machine.vi"("State(s) in (\"\")"=w222) -> ("States Out"=w221:string)  [unwired: 14 in]
      }
      frame "Events: Register" {
        n93 = call "Read stop event.vi"("GUI in"=w225) -> ("cmd event"=w223:refnum<user-event>, "stop event"=w224:refnum<user-event>)  [unwired: 8 in, 1 out]
        n94 = register-events(error in=w226, w224, w223) -> (reference out=w228:refnum<event-registration>, error out=w227:errorcluster)  [unwired: 1 in]
      }
      frame "Events: Unregister" {
        # "Do not put any code in this frame.\n(It is a separator no-op. You can make a copy of this frame to create a new UI frame)"
        n95 = Unregister For Events(event registration refnum=w233, error in=w232) -> (error out=w231:errorcluster)
        n96 = call <vilib>:"Add State(s) to Queue__JKI_lib_State_Machine.vi"("State(s) in (\"\")"=w236) -> ("States Out"=w235:string)  [unwired: 14 in]
      }
      frame "---------- UI ----------" {
        # "Do not put any code in this frame.\n(It is a separator no-op. You can make a copy of this frame to create a new UI frame)"
        n97 = call <vilib>:"Add State(s) to Queue__JKI_lib_State_Machine.vi"("State(s) in (\"\")"=w241) -> ("States Out"=w240:string)  [unwired: 14 in]
      }
      frame "UI: Initialize" {
      }
      frame "UI: Cursor Set" {
        # "Argument"
        # "Set and Unset Cursor Busy.\n(Usage: \"UI: Cursor Set >> Busy|Idle\")"
        n98 = case shown="\"Idle\", Default" w247 {
          tunnel: w249 -> [w254 w256]
          tunnel: [w253 w255] -> w248
          frame "Idle", Default {
            n99 = call <vilib>:"Unset Busy.vi"("error in (no error)"=w254) -> ("error out"=w253:errorcluster)  [unwired: 10 in]
          }
          frame "Busy" {
            n100 = call <vilib>:"Set Busy.vi"("error in (no error)"=w256) -> ("error out"=w255:errorcluster)  [unwired: 9 in, 1 out]
          }
        }
        n101 = call <vilib>:"Add State(s) to Queue__JKI_lib_State_Machine.vi"("State(s) in (\"\")"=w252) -> ("States Out"=w251:string)  [unwired: 14 in]
      }
      frame "UI: Front Panel State" {
        # "Argument"
        # "Set Front Panel Open or Closed\n(Usage: \"UI: Front Panel State >> Open|Close\")"
        n102 = Unbundle By Name(w260) -> ("Core.Current VI Reference"=w259:refnum<vi>)
        n103 = case shown="\"Minimize\", \"Minimized\"" w258 {
          tunnel: w262 -> [w270 w285 w296 w309 w322]
          tunnel: [w272 w286 w298 w311 w324] -> w261
          tunnel: w259 -> [w271 w283 w297 w310 w323]
          frame "Open", "Standard", Default {
            w265 = T6."Standard" ("State")
            n104 = property class="VI"(reference=w271, error in=w270) -> (reference out=w268:refnum<vi>, error out=w269:errorcluster, "FP.State"=w267:T6)
            n105 = Not Equal?(x=w267, y=w265) -> (x != y?=w266:bool)
            n106 = case shown="True" w266 {
              tunnel: [w276 w278] -> w272
              tunnel: w269 -> [w275 w278]
              tunnel: w268 -> [w274 _]
              tunnel: w265 -> [w273 _]
              frame True {
                n107 = invoke class="VI" method="FP.Open"(reference=w274, error in=w275, "Activate"=TRUE, "State"=w273) -> (error out=w276:errorcluster)  [unwired: 1 in, 4 out]
              }
              frame False {
              }
            }
          }
          frame "Close", "Closed" {
            n108 = property class="VI"(reference=w283, error in=w285) -> (reference out=w282:refnum<vi>, error out=w284:errorcluster, "FP.State"=w280:T6)
            n109 = Not Equal?(x=w280, y=T6."Closed" ("Front Panel Window:State")) -> (x != y?=w279:bool)
            n110 = case shown="True" w279 {
              tunnel: [w287 w290] -> w286
              tunnel: w284 -> [w287 w289]
              tunnel: w282 -> [_ w288]
              frame False {
              }
              frame True {
                n111 = invoke class="VI" method="FP.Close"(reference=w288, error in=w289) -> (error out=w290:errorcluster)  [unwired: 1 in, 2 out]
              }
            }
          }
          frame "Hidden", "Hide" {
            w291 = T6."Hidden" ("State")
            n112 = property class="VI"(reference=w297, error in=w296) -> (reference out=w294:refnum<vi>, error out=w295:errorcluster, "FP.State"=w293:T6)
            n113 = Not Equal?(x=w293, y=w291) -> (x != y?=w292:bool)
            n114 = case shown="True" w292 {
              tunnel: [w302 w303] -> w298
              tunnel: w295 -> [w301 w303]
              tunnel: w294 -> [w300 _]
              tunnel: w291 -> [w299 _]
              frame True {
                n115 = invoke class="VI" method="FP.Open"(reference=w300, error in=w301, "State"=w299) -> (error out=w302:errorcluster)  [unwired: 2 in, 4 out]
              }
              frame False {
              }
            }
          }
          frame "Minimize", "Minimized" {
            w304 = T6."Minimized" ("State")
            n116 = property class="VI"(reference=w310, error in=w309) -> (reference out=w307:refnum<vi>, error out=w308:errorcluster, "FP.State"=w306:T6)
            n117 = Not Equal?(x=w306, y=w304) -> (x != y?=w305:bool)
            n118 = case shown="True" w305 {
              tunnel: [w315 w316] -> w311
              tunnel: w308 -> [w314 w316]
              tunnel: w307 -> [w313 _]
              tunnel: w304 -> [w312 _]
              frame True {
                n119 = invoke class="VI" method="FP.Open"(reference=w313, error in=w314, "State"=w312) -> (error out=w315:errorcluster)  [unwired: 2 in, 4 out]
              }
              frame False {
              }
            }
          }
          frame "Maximize", "Maximized" {
            w317 = T6."Maximized" ("State")
            n120 = property class="VI"(reference=w323, error in=w322) -> (reference out=w320:refnum<vi>, error out=w321:errorcluster, "FP.State"=w319:T6)
            n121 = Not Equal?(x=w319, y=w317) -> (x != y?=w318:bool)
            n122 = case shown="True" w318 {
              tunnel: [w328 w329] -> w324
              tunnel: w321 -> [w327 w329]
              tunnel: w320 -> [w326 _]
              tunnel: w317 -> [w325 _]
              frame True {
                n123 = invoke class="VI" method="FP.Open"(reference=w326, error in=w327, "State"=w325) -> (error out=w328:errorcluster)  [unwired: 2 in, 4 out]
              }
              frame False {
              }
            }
          }
        }
        n124 = call <vilib>:"Add State(s) to Queue__JKI_lib_State_Machine.vi"("State(s) in (\"\")"=w264) -> ("States Out"=w263:string)  [unwired: 14 in]
      }
      frame "---------- Macro ----------" {
        # "Do not put any code in this frame.\n(It is a separator no-op. You can make a copy of this frame to create a new Macro frame)"
        n125 = call <vilib>:"Add State(s) to Queue__JKI_lib_State_Machine.vi"("State(s) in (\"\")"=w334) -> ("States Out"=w333:string)  [unwired: 14 in]
      }
      frame "Macro: Initialize" {
        n126 = call <vilib>:"Add State(s) to Queue__JKI_lib_State_Machine.vi"("State(s) in Front (\"\")"="Data: Initialize\nInitialize Core Data\nEvents: Register\nUI: Initialize\n// UI: Front Panel State >> Open\n\n\nAction: Read Config", "State(s) in (\"\")"=w340) -> ("States Out"=w339:string)  [unwired: 13 in]
      }
      frame "Macro: Update" {
        n127 = call <vilib>:"Add State(s) to Queue__JKI_lib_State_Machine.vi"("State(s) in Front (\"\")"="Action: Write Config", "State(s) in (\"\")"=w346) -> ("States Out"=w345:string)  [unwired: 13 in]
      }
      frame "Macro: Exit" {
        # "Exit Macro\n(This is called once, when the VI exits)"
        n128 = Unbundle By Name(w355) -> ("Core.Close Panel on Exit?"=w354:bool)
        n129 = Select(t="UI: Front Panel State >> Close", s=w354, f="") -> (s? t:f=w351:string)
        n130 = call <vilib>:"Add State(s) to Queue__JKI_lib_State_Machine.vi"("State(s) in Front (\"\")"="Action: Write Config", "State(s) in (\"\")"=w351, "State(s) at Back (\"\")"="Data: Cleanup\nEvents: Unregister\nExit") -> ("States Out"=w349:string)  [unwired: 12 in]
        n131 = call <vilib>:"Add State(s) to Queue__JKI_lib_State_Machine.vi"("State(s) in Front (\"\")"=w349, "State(s) in (\"\")"=w358) -> ("States Out"=w357:string)  [unwired: 13 in]
      }
      frame "---------- Action ----------" {
      }
      frame "Action: Read Config" {
        n132 = call "Read SVW.vi"("GUI in"=w364) -> ("SharedVariableWrapper.lvclass"=w363:refnum<class "SharedVariableWrapper.lvclass">)  [unwired: 10 in]
        n133 = in-place {
          in-place-border: w369 -> [w375]
          in-place-border: [w374] -> w368
          in-place-border: w363 -> [w376]
          n134 = in-place-cluster #1(w367) -> ("satting name"=w372:string, "Needle Valve Settings"=w373:T1)
          n135 = call "Read.vim"("SharedVariableWrapper in"=w376, "name"=w372, "DataType"=w373, "error in (no error)"=w375) -> ("data out"=w371:T1, "error out"=w374:errorcluster)  [unwired: 5 in, 5 out]
          n136 = local write "Needle Valve Settings"(w371) -> ()
          n137 = in-place-cluster #1("satting name"=w372, "Needle Valve Settings"=w371) -> (w366:T9)
        }
      }
      frame "Action: Write Config" {
        n138 = Unbundle By Name(w380) -> ("Needle Valve Settings"=w379:T1)
        n139 = Unbundle By Name(w380) -> ("amc"=w387:refnum<class "MessageAMC.lvclass">)
        n140 = call "Read name.vi"("GUI in"=w377) -> ("name"=w378:string)  [unwired: 9 in, 1 out]
        n141 = call "Read SVW.vi"("GUI in"=w377) -> ("SharedVariableWrapper.lvclass"=w390:refnum<class "SharedVariableWrapper.lvclass">)  [unwired: 10 in]
        n142 = call "ReadConfig.vi"("SharedVariableWrapper in"=w390) -> ("config"=w389:T8)  [unwired: 12 in, 2 out]
        n143 = Unbundle By Name(w389) -> ("ip"=w388:string)
        n144 = call "SendNetworkVariant.vi"("reference in"=w387, "receiver process"=w378, "receiver host"=w388, "receiver port (0)"=u16 54321, "name"="SET_SETTINGS", "data"=w379, "timeout (25000 ms)"=1000, "error in (no error)"=w382) -> ("error out"=w384:errorcluster)  [unwired: 5 in, 2 out]
        n145 = call <vilib>:"Simple Error Handler.vi"("error in (no error)"=w384) -> ("error out"=w381:errorcluster)  [unwired: 4 in, 4 out]
      }
    }
  }
  n146 = call "Read name.vi"("GUI in"=w4) -> ("name"=w2:string)  [unwired: 9 in, 1 out]
  n147 = call "Read SVW.vi"("GUI in"=w4) -> ("SharedVariableWrapper.lvclass"=w6:refnum<class "SharedVariableWrapper.lvclass">)  [unwired: 10 in]
  n148 = Concatenate Strings(w2, "DATA" ("name")) -> (w1:string)
  n149 = property on="Engine State" class="Ring (strict)"() -> ("Strings []"=w5:string[])  [unwired: 2 in, 2 out]
  n150 = while {
    tunnel: w6 -> [w399]
    tunnel: w5 -> [w394]
    tunnel: w1 -> [w393]
    stop <- "stop" stop-if-true
    n151 = stacked-sequence {
      tunnel: w399 -> [w403 w426]
      tunnel: [w419 _] -> w397
      tunnel: [_ w423] -> w398
      tunnel: w394 -> [w406 _]
      tunnel: w393 -> [w402 _]
      frame #0 {
        n152 = call "Read.vim"("SharedVariableWrapper in"=w403, "name"=w402, "DataType"=T11 {"Engine State"=8, "StateValveModbus"=enum."IDLE", "Alarms"={"OL"=FALSE, "TF"=FALSE, "STL"=FALSE, "OCP"=FALSE, "CPUV"=FALSE, "UVLO"=FALSE, "SPI_ERROR"=FALSE, "Fault"=FALSE, "OL 2"=FALSE, "TF 2"=FALSE, "STL 2"=FALSE, "OCP 2"=FALSE, "CPUV 2"=FALSE, "UVLO 2"=FALSE, "reserved"=TRUE, "InitDone"=TRUE}, "RAW Possition"=124110, "Angele"=0.0, "Step"=0, "Encoder"=0, "Kinematic"={"ACC Steps Per Sec^2"=100, "DEC Steps Per Sec^2"=100, "Min Velosity Step Per Sec"=100, "Max Velosity Step Per Sec"=200, "MicroStep"=16}, "Limits"={"Fault 2 Switch"=FALSE, "Fault 1 Switch"=FALSE, "Center(Home)"=FALSE, "Lower Limit"=FALSE, "Upper Limit"=FALSE}} ("NVM Data")) -> ("data out"=w417:T11, "error out"=w419:errorcluster)  [unwired: 6 in, 5 out]
        n153 = Unbundle By Name(w417) -> ("Alarms"=→"Alarms":T5, "Engine State"=w405:T3, "StateValveModbus"=w407:T12, "Angele"=→"Waveform Chart - Dark 3":dbl, "Step"=→"step":i32, "Encoder"=→"encoder":i32, "Kinematic"=→"Kinematic":T2)  [unwired: 1 out]
        n154 = Index Array(array=w406, index=w405) -> (element=w404:string)
        n155 = Format Into String(format string="DRIVER STATE: %s", w404) -> (resulting string=→"String":string)  [unwired: 2 in, 1 out]
        n156 = Format Into String(format string="VALVE STATE: %s ", w407) -> (resulting string=→"String 2":string)  [unwired: 2 in, 1 out]
      }
      frame #1 {
        n157 = call "Read.vim"("SharedVariableWrapper in"=w426, "name"="DO_ARRAY_OUT", "DataType"=bool[] []) -> ("data out"=w422:bool[], "error out"=w423:errorcluster)  [unwired: 6 in, 5 out]
        n158 = Index Array(array=w422, index=19) -> (element=→"DO 19":bool)
      }
    }
    n159 = Merge Errors(w398, w397) -> (w396:errorcluster)
    n160 = Wait Until Next ms Multiple(millisecond multiple=u32 100) -> ()  [unwired: 1 out]
    n161 = Unbundle By Name(w396) -> ("status"=→"Connect":bool)
  }
  n162 = flat-sequence {
    tunnel: w11 -> [w428]
    frame #0 {
      n163 = local write "stop"(TRUE ("stop")) -> ()
      "error out" <- w428
    }
  }
